vi "Free Known Host.vi"(8 "error in (no error)":errorcluster, 11 "known host":T1) -> (0 "error out":errorcluster)   [LabVIEW 2013, in "libssh2.lvlib"]
doc: "Releases all ressources associated with <B>known host</B>."
uses:
  libssh2.lvlib
  Known Host Refnum.ctl
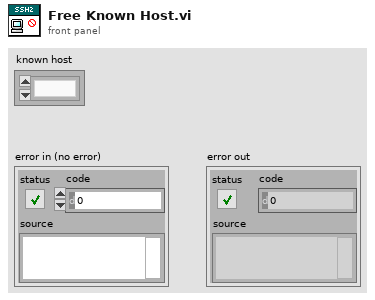
[diagram p1: front panel]
types:
  T1 = typedef "libssh2.lvlib/Known Host Refnum.ctl" = refnum<k1>
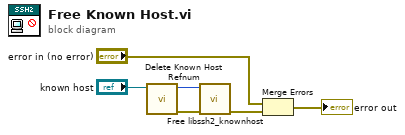
[diagram p0: block diagram]
diagram:
  n1 = call "Delete Known Host Refnum.vi"("Host"="known host") -> ("error out"=w6:errorcluster, "libssh2_knownhost*"=w5:u64)  [unwired: 9 in]
  n2 = call "Free libssh2_knownhost.vi"("error in (no error)"=w6, "libssh2_knownhost*"=w5) -> ("error out"=w3:errorcluster)  [unwired: 9 in]
  n3 = Merge Errors("error in (no error)", w3) -> (→"error out":errorcluster)
